vi "LIA.SR810.GetResource.vi"(8 "error in (no error)":errorcluster, 11 "LIA.SR810 in":refnum<class "LIA.SR810.lvclass">) -> (0 "error out":errorcluster, 2 "Resource":T1, 3 "LIA.SR810 out":refnum<class "LIA.SR810.lvclass">)   [LabVIEW 2017, in "LIA.SR810.lvclass"]
uses:
  LIA.SR810.lvclass
  LIA.SR810.lvclass/LIA.SR810.ctl
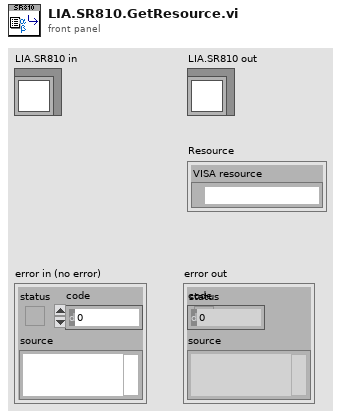
[diagram p1: front panel]
types:
  T1 = cluster{"VISA resource":refnum<visa-resource-name>}
  T2 = typedef "LIA.SR810.lvclass/PrivateData--Ref.ctl" = refnum<data-value>
  T3 = typedef "LIA.SR810.lvclass/PrivateData--Cluster.ctl" = cluster{"Resource":cluster{"VISA resource":refnum<visa-resource-name>}}
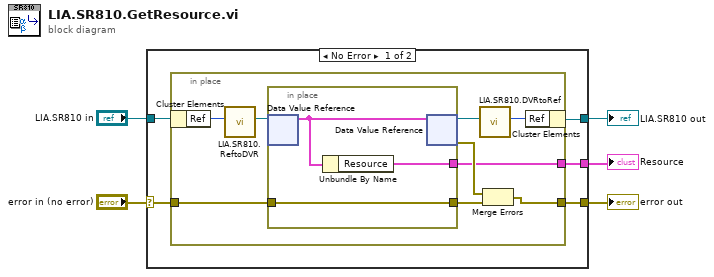
[diagram p0: block diagram]
diagram:
  n1 = case shown="No Error" "error in (no error)" {
    selector: "error in (no error)" -> [w8 w24]
    tunnel: [w7 w24] -> w4
    tunnel: [w9 w23] -> w2
    tunnel: "LIA.SR810 in" -> [w10 w23]
    tunnel: [w6 _] -> w1
    frame No Error {
      n2 = in-place {
        in-place-border: w8 -> [w15]
        in-place-border: [w12] -> w7
        in-place-border: [w11] -> w6
        n3 = in-place-cluster #1(w10) -> ("Ref"=w19:u32)
        n4 = call "LIA.SR810.ReftoDVR.vi"("Ref"=w19) -> ("Ref"=w16:T2)  [unwired: 10 in]
        n5 = in-place {
          in-place-border: w15 -> [w22]
          in-place-border: [w22] -> w13
          in-place-border: [w20] -> w11
          n6 = in-place-dvr #2(w16) -> (w21:T3)  [unwired: 1 out]
          n7 = Unbundle By Name(w21) -> ("Resource"=w20:T1)
          n8 = in-place-dvr #2(w21) -> (w17:T2, w14:errorcluster)
        }
        n9 = call "LIA.SR810.DVRtoRef.vi"("Ref"=w17) -> ("Ref"=w18:u32)  [unwired: 10 in]
        n10 = Merge Errors(w14, w13) -> (w12:errorcluster)
        n11 = in-place-cluster #1("Ref"=w18) -> (w9:refnum<class "LIA.SR810.lvclass">)
      }
    }
    frame Error {
    }
  }
  "error out" <- w4
  "LIA.SR810 out" <- w2
  "Resource" <- w1
